vi "Read ARN.vi"(8 "error in (no error)":errorcluster, 11 "ARN":refnum<class "ARN.lvclass">) -> (0 "error out":errorcluster, 2 "Amazon Resource Name":string, 3 "ARN out":refnum<class "ARN.lvclass">)   [LabVIEW 2015, in "NI_AWS_Core.lvlib" / "ARN.lvclass"]
uses:
  ARN.lvclass
  ARN.lvclass/ARN.ctl
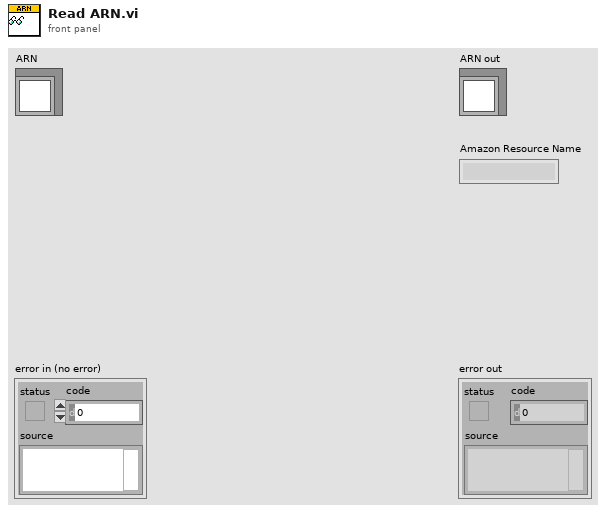
[diagram p1: front panel]
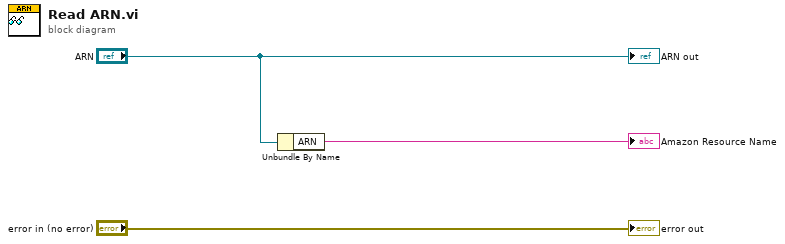
[diagram p0: block diagram]
diagram:
  n1 = Unbundle By Name("ARN") -> ("ARN"=→"Amazon Resource Name":string)
  "error out" <- "error in (no error)"
  "ARN out" <- "ARN"
